vi "SVD data.vi"(1 "Data":dbl[][](array[numeric])) -> (0 "Data out":dbl[][](array[numeric]))   [LabVIEW 2009]
uses:
  <vilib>/Math Plots/3D Math Plots/3D Scatter/3D Scatter XCtrl/3D Scatter.xctl
  <vilib>/Analysis/7linalg.llb/Eigenvalue and Vectors Output Option.ctl
  <vilib>/Math Plots/3D Math Plots/3D Scatter/3D Scatter Datatype/Public/Plot Helper (Vector).vi
  <vilib>/Analysis/Matrix/Numeric/Conversions/Matrix To Array - RM.vi
  <vilib>/Analysis/baseanly.llb/Real A x B.vi
  <vilib>/Analysis/Matrix/Numeric/Complex/Complex To Cartesian - CM.vi
  <vilib>/Analysis/7linalg.llb/Real Eigenvalues and Vectors.vi
  <vilib>/Analysis/7linalg.llb/Real Transpose Matrix.vi
  <vilib>/Analysis/Matrix/Numeric/Conversions/Array To Matrix - RA2.vi
  <vilib>/Analysis/Matrix/NI_Matrix.lvlib
  <vilib>/Analysis/NI_AALPro.lvlib
  <vilib>/Analysis/NI_AALBase.lvlib
  <vilib>/Math Plots/3D Math Plots/3D Scatter/3D Scatter Datatype/3D Scatter Datatype.lvclass
panel:
  out "pre-transformed":refnum<class "3D Plot Datatype.lvclass">[](xcontrol)
  out "Transformed data":refnum<class "3D Plot Datatype.lvclass">[](xcontrol)
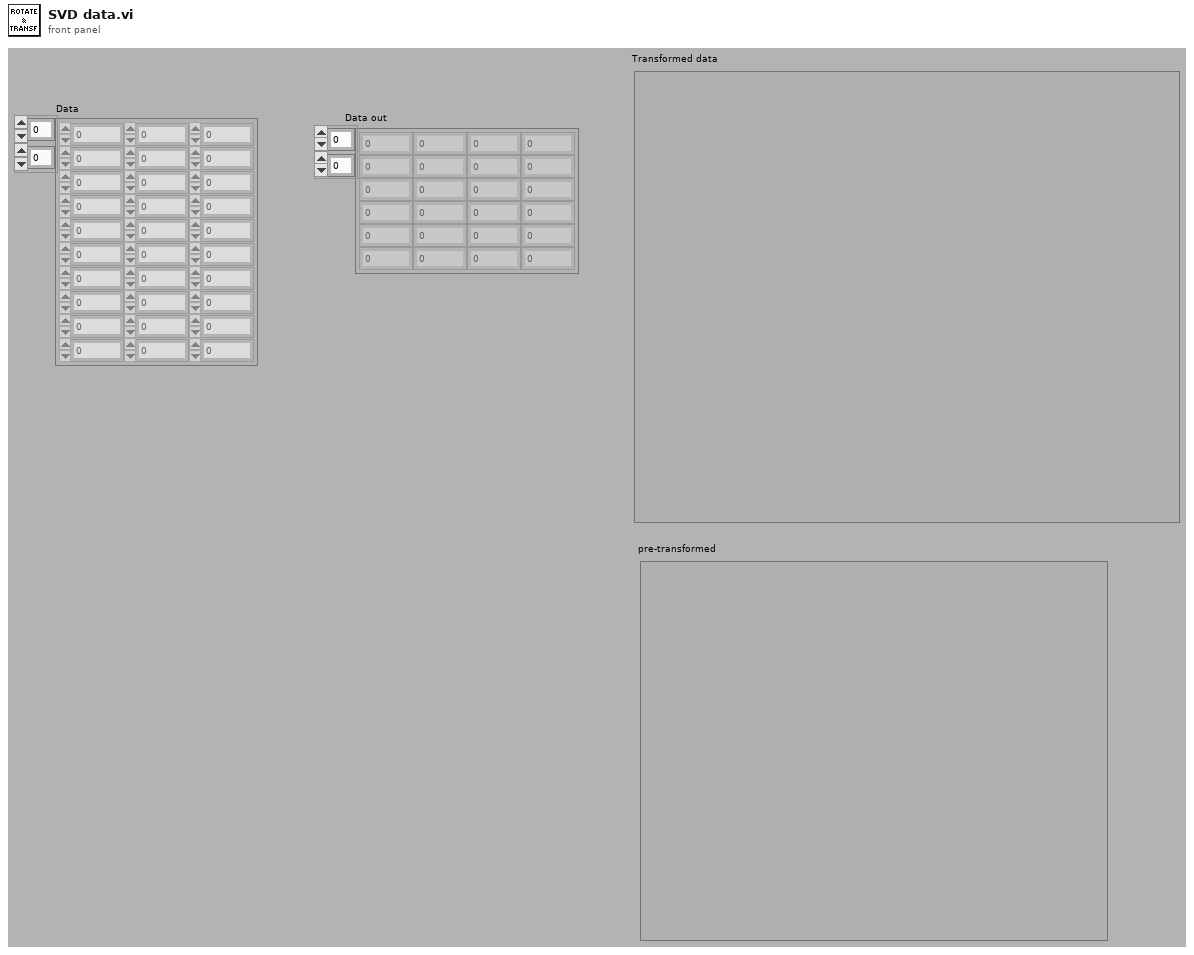
[diagram p1: front panel]
types:
  T1 = typedef "NI_AALPro.lvlib/Eigenvalue and Vectors Output Option.ctl" = i32
  T2 = typedef "NI_Matrix.lvlib/RealMatrix.ctl" = dbl[][]
  T3 = typedef "NI_Matrix.lvlib/ComplexMatrix.ctl" = cdb[][]
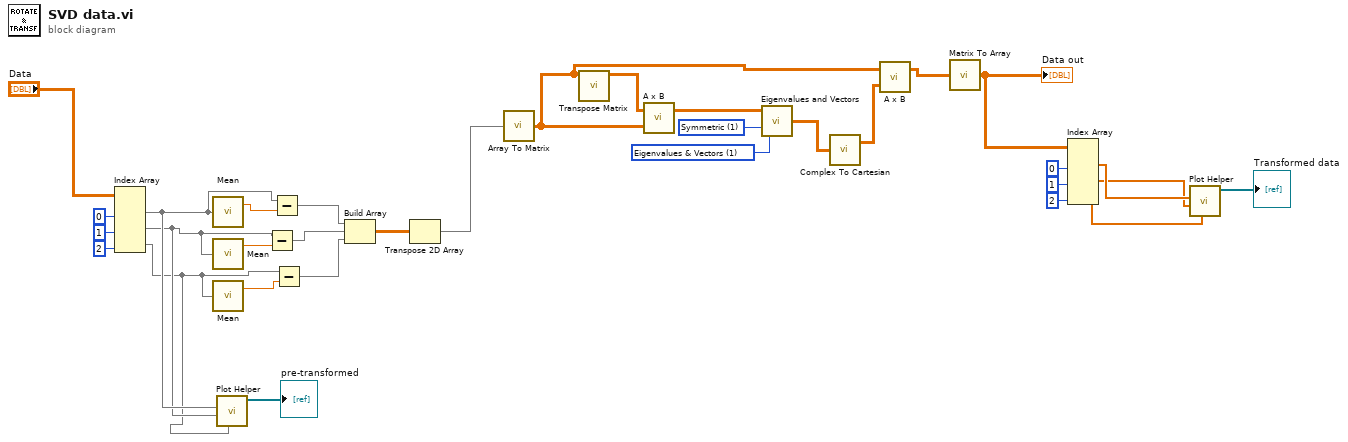
[diagram p0: block diagram]
diagram:
  w29 = T1 1 items=["Eigenvalues", "Eigenvalues & Vectors"] ("output option")
  w30 = 1 items=["General", "Symmetric"] ("matrix type")
  n1 = Index Array(array="Data", index (col) #1=0 ("disabled index (col)"), index (col) #2=1 ("index (col)"), index (col) #3=2 ("index (col)")) -> (element #1=w3:dbl[], element #2=w2:dbl[], element #3=w1:dbl[])  [unwired: 3 in]
  n2 = call <vilib>:"Mean.vi"("X"=w3) -> ("mean"=w21:dbl)  [unwired: 1 out]
  n3 = call <vilib>:"Mean.vi"("X"=w2) -> ("mean"=w22:dbl)  [unwired: 1 out]
  n4 = call <vilib>:"Mean.vi"("X"=w1) -> ("mean"=w24:dbl)  [unwired: 1 out]
  n5 = call-poly <vilib>:"Plot Helper.vi"("z vector"=w1, "y vector"=w2, "x vector"=w3) -> ("3D Plot lvclass Array out"=→"pre-transformed":refnum<class "3D Plot Datatype.lvclass">[])  [unwired: 3 in, 5 out]
  n6 = Subtract(x=w2, y=w22) -> (x-y=w19:dbl[])
  n7 = Subtract(x=w3, y=w21) -> (x-y=w18:dbl[])
  n8 = Subtract(x=w1, y=w24) -> (x-y=w20:dbl[])
  n9 = Build Array(w18, w19, w20) -> (w23:dbl[][])
  n10 = Transpose 2D Array(2D array=w23) -> (transposed array=w17:dbl[][])
  n11 = call-poly <vilib>:"Array To Matrix.vi"("Real 2D Array"=w17) -> ("Real Matrix"=w14:T2)
  n12 = call-poly <vilib>:"Transpose Matrix.vi"("Input Matrix"=w14) -> ("Matrix Transpose"=w32:T2)  [unwired: 9 in, 1 out]
  n13 = call-poly <vilib>:"A x B.vi"("B"=w14, "A"=w32) -> ("A x B"=w31:T2)  [unwired: 1 out]
  n14 = call-poly <vilib>:"Eigenvalues and Vectors.vi"("output option"=w29, "matrix type"=w30, "Input Matrix"=w31) -> ("Eigenvectors"=w16:T3)  [unwired: 2 out]
  n15 = call-poly <vilib>:"Complex To Cartesian.vi"("Complex Matrix R + Ii"=w16) -> ("Real Matrix R"=w13:T2)  [unwired: 1 out]
  n16 = call-poly <vilib>:"A x B.vi"("B"=w13, "A"=w14) -> ("A x B"=w15:T2)  [unwired: 1 out]
  n17 = call-poly <vilib>:"Matrix To Array.vi"("Real Matrix"=w15) -> ("Real 2D Array"=w9:dbl[][])
  "Data out" <- w9
  n18 = Index Array(array=w9, index (col) #1=0 ("disabled index (col)"), index (col) #2=1 ("index (col)"), index (col) #3=2 ("index (col)")) -> (element #1=w7:dbl[], element #2=w6:dbl[], element #3=w5:dbl[])  [unwired: 3 in]
  n19 = call-poly <vilib>:"Plot Helper.vi"("z vector"=w5, "y vector"=w6, "x vector"=w7) -> ("3D Plot lvclass Array out"=→"Transformed data":refnum<class "3D Plot Datatype.lvclass">[])  [unwired: 3 in, 5 out]
